vi "sub parse frame o.vi"(8 "error in (no error)":errorcluster, 11 "<o> String":string="   <o kind 1 x 46 y 75 action 70 oid 204 o>") -> (0 "error out":errorcluster, 3 "<o> data":T1)   [LabVIEW 2018, in "Data Parser.lvclass"]
uses:
  Data Parser.lvclass
  frame o data.ctl
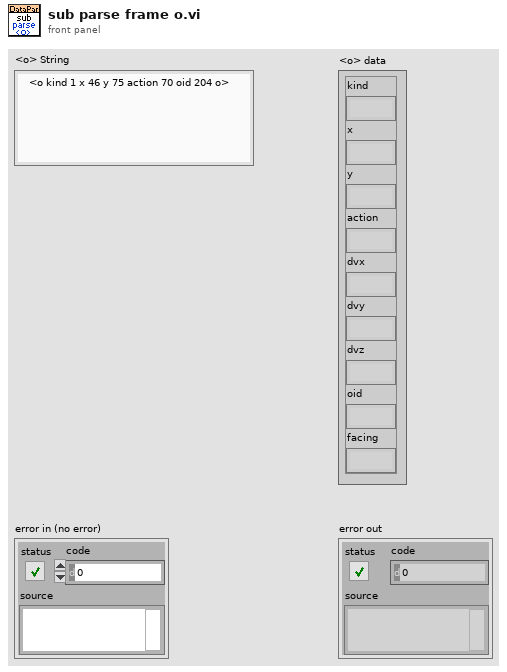
[diagram p1: front panel]
types:
  T1 = typedef "Data Parser.lvclass/frame o data.ctl" = cluster{"kind":string, "x":string, "y":string, "action":string, "dvx":string, "dvy":string, "dvz":string, "oid":string, "facing":string}
  T2 = cluster{"[0]":string, "[1]":string, "[2]":string, "[3]":string, "[4]":string, "[5]":string, "[6]":string, "[7]":string, "[8]":string}
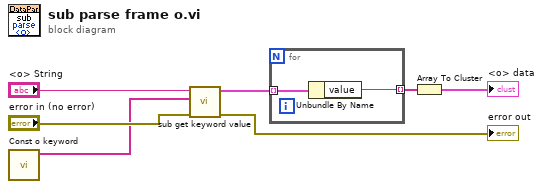
[diagram p0: block diagram]
diagram:
  n1 = call "Const o keyword.vi"() -> ("Const o keyword"=w1:string[])  [unwired: 11 in]
  n2 = call "sub get keyword value.vi"("error in"="error in (no error)", "keyword"=w1, "string"="<o> String") -> ("error out"=→"error out":errorcluster, "matched pairs (all)"=w4:cluster{"keyword":string, "value":string}[])  [unwired: 5 in, 2 out]
  n3 = for {
    tunnel: w4 -> [w9] mode=indexing
    tunnel: [w8] -> w3 mode=indexing
    n4 = Unbundle By Name(w9) -> ("value"=w8:string)
  }
  n5 = Array To Cluster(array=w3) -> (cluster=→"<o> data":T2)
